vi "Teleop.vi"(10 "Match Info":T1={"Autonomous Elapsed Seconds"=0.0, "TeleOp Elapsed Seconds"=0.0, "Disabled Elapsed Seconds"=0.0, "Visited Autonomous"=FALSE, "Visited TeleOp"=FALSE, "Visited Disabled"=FALSE, "Autonomous Settings"={"Autonomous Style"=enum."Independent", "VI Refnum"=refnum}}, 11 "Call Context":T2) -> ()   [LabVIEW 2013]
doc: "This VI is called for each TeleOp packet received from the DS where the robot is not disabled. It is often used to read from the joysticks and update I/O or to update setpoints for timed control loops. It should complete and return within 20 milliseconds or it may miss DS packets."
uses:
  <vilib>/Rock Robotics/WPI/DriverStation/WPI_DriverStationDerivedRobotMode.ctl
  <vilib>/Rock Robotics/WPI/DriverStation/WPI_DriverStationMatch Info.ctl
  <vilib>/Rock Robotics/WPI/Solenoid/WPI_SolenoidValue.ctl
  Robot Global Data.vi
  <vilib>/Rock Robotics/WPI/RobotDrive/WPI_RobotDriveArcadeDrive_Standard(NoSaturation).vi
  <vilib>/Rock Robotics/WPI/Solenoid/WPI_SolenoidSetEnum.vi
  <vilib>/Rock Robotics/WPI/Joystick/WPI_JoystickGetSetRefNum.vi
  <vilib>/Rock Robotics/WPI/RobotDrive/WPI_RobotDriveGetSetRefNum.vi
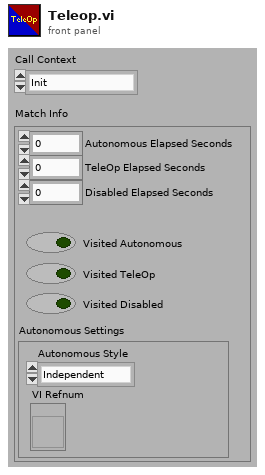
[diagram p1: front panel]
types:
  T1 = typedef "WPI_DriverStationMatch Info.ctl" = cluster{"Autonomous Elapsed Seconds":dbl, "TeleOp Elapsed Seconds":dbl, "Disabled Elapsed Seconds":dbl, "Visited Autonomous":bool, "Visited TeleOp":bool, "Visited Disabled":bool, "Autonomous Settings":cluster{"Autonomous Style":enum16{"Iterative", "Independent"}, "VI Refnum":refnum<vi>}}
  T2 = typedef "WPI_DriverStationDerivedRobotMode.ctl" = enum16{"Init", "Execute", "Stop"}
  T3 = typedef "WPI_SolenoidValue.ctl" = enum16{"Off", "On", "Forward", "Reverse"}
  T4 = typedef "WPI_JoystickDevRef.ctl" = cluster{"Device":T5}
  T5 = typedef "WPI_JoystickDeviceEnum.ctl" = enum16{"USB 1", "USB 2", "USB 3", "USB 4", "Kinect 1", "Kinect 2"}
  T6 = typedef "WPI_MotorControlDeviceRef.ctl" = cluster{"DeviceStatus":errorcluster, "Type":enum16{"PWM", "CAN"}, "PWM":cluster{"Digital Module":T7, "PWM Channel":T8, "DeadBand":T9}, "CAN":cluster{"Device Number":u8, "Control Mode":T10, "Semaphore":T11, "Max Vout":dbl}, "Invert":bool, "TransformRef":T12, "InvTransformRef":T12}
  T7 = typedef "FPGA_TypedefDigitalModule.ctl" = enum16{"Digital Module 1", "Digital Module 2"}
  T8 = typedef "FPGA_DIOPWMChannel.ctl" = enum8{"PWM 1", "PWM 2", "PWM 3", "PWM 4", "PWM 5", "PWM 6", "PWM 7", "PWM 8", "PWM 9", "PWM 10", "Invalid"}
  T9 = typedef "WPI_PWMDeadband.ctl" = cluster{"Name":string, "maxPositivePwm":i32, "minPositivePwm":i32, "centerPwm":i32, "maxNegativePwm":i32, "minNegativePwm":i32, "angularRange":u16}
  T10 = typedef "WPI_CANJaguar_ControlMode.ctl" = enum8{"Percent VBus", "Current", "Speed", "Position", "Voltage"}
  T11 = typedef "Semaphore RefNum" = refnum<k1>
  T12 = typedef "WPI_PWMTransform_ConPane.ctl" = refnum<vi>
  T13 = typedef "WPI_JoystickButtonState.ctl" = cluster{"Button 1":bool, "Button 2":bool, "Button 3":bool, "Button 4":bool, "Button 5":bool, "Button 6":bool, "Button 7":bool, "Button 8":bool, "Button 9":bool, "Button 10":bool, "Button 11":bool, "Button 12":bool}
  T14 = cluster{"axis 1 (x)":dbl, "axis 2 (y)":dbl, "axis 3 (throttle)":dbl, "axis 4":dbl, "axis 5":dbl, "axis 6":dbl}
  T15 = typedef "WPI_SolenoidDevRef.ctl" = cluster{"DevStatus":errorcluster, "Solenoid Module":T16, "Forward Solenoid Channel":T17, "Reverse Solenoid Channel":T17}
  T16 = typedef "FPGA_TypedefSolenoidModule.ctl" = enum16{"Solenoid Module 1", "Solenoid Module 2"}
  T17 = typedef "WPI_SolenoidChannel.ctl" = enum8{"Solenoid 1", "Solenoid 2", "Solenoid 3", "Solenoid 4", "Solenoid 5", "Solenoid 6", "Solenoid 7", "Solenoid 8", "Invalid"}
  T18 = typedef "WPI_RobotDriveDevRef.ctl" = cluster{"DevStatus":errorcluster, "Motors[]":T6[], "Square Inputs":bool, "Max Output":dbl, "Isochronous":bool}
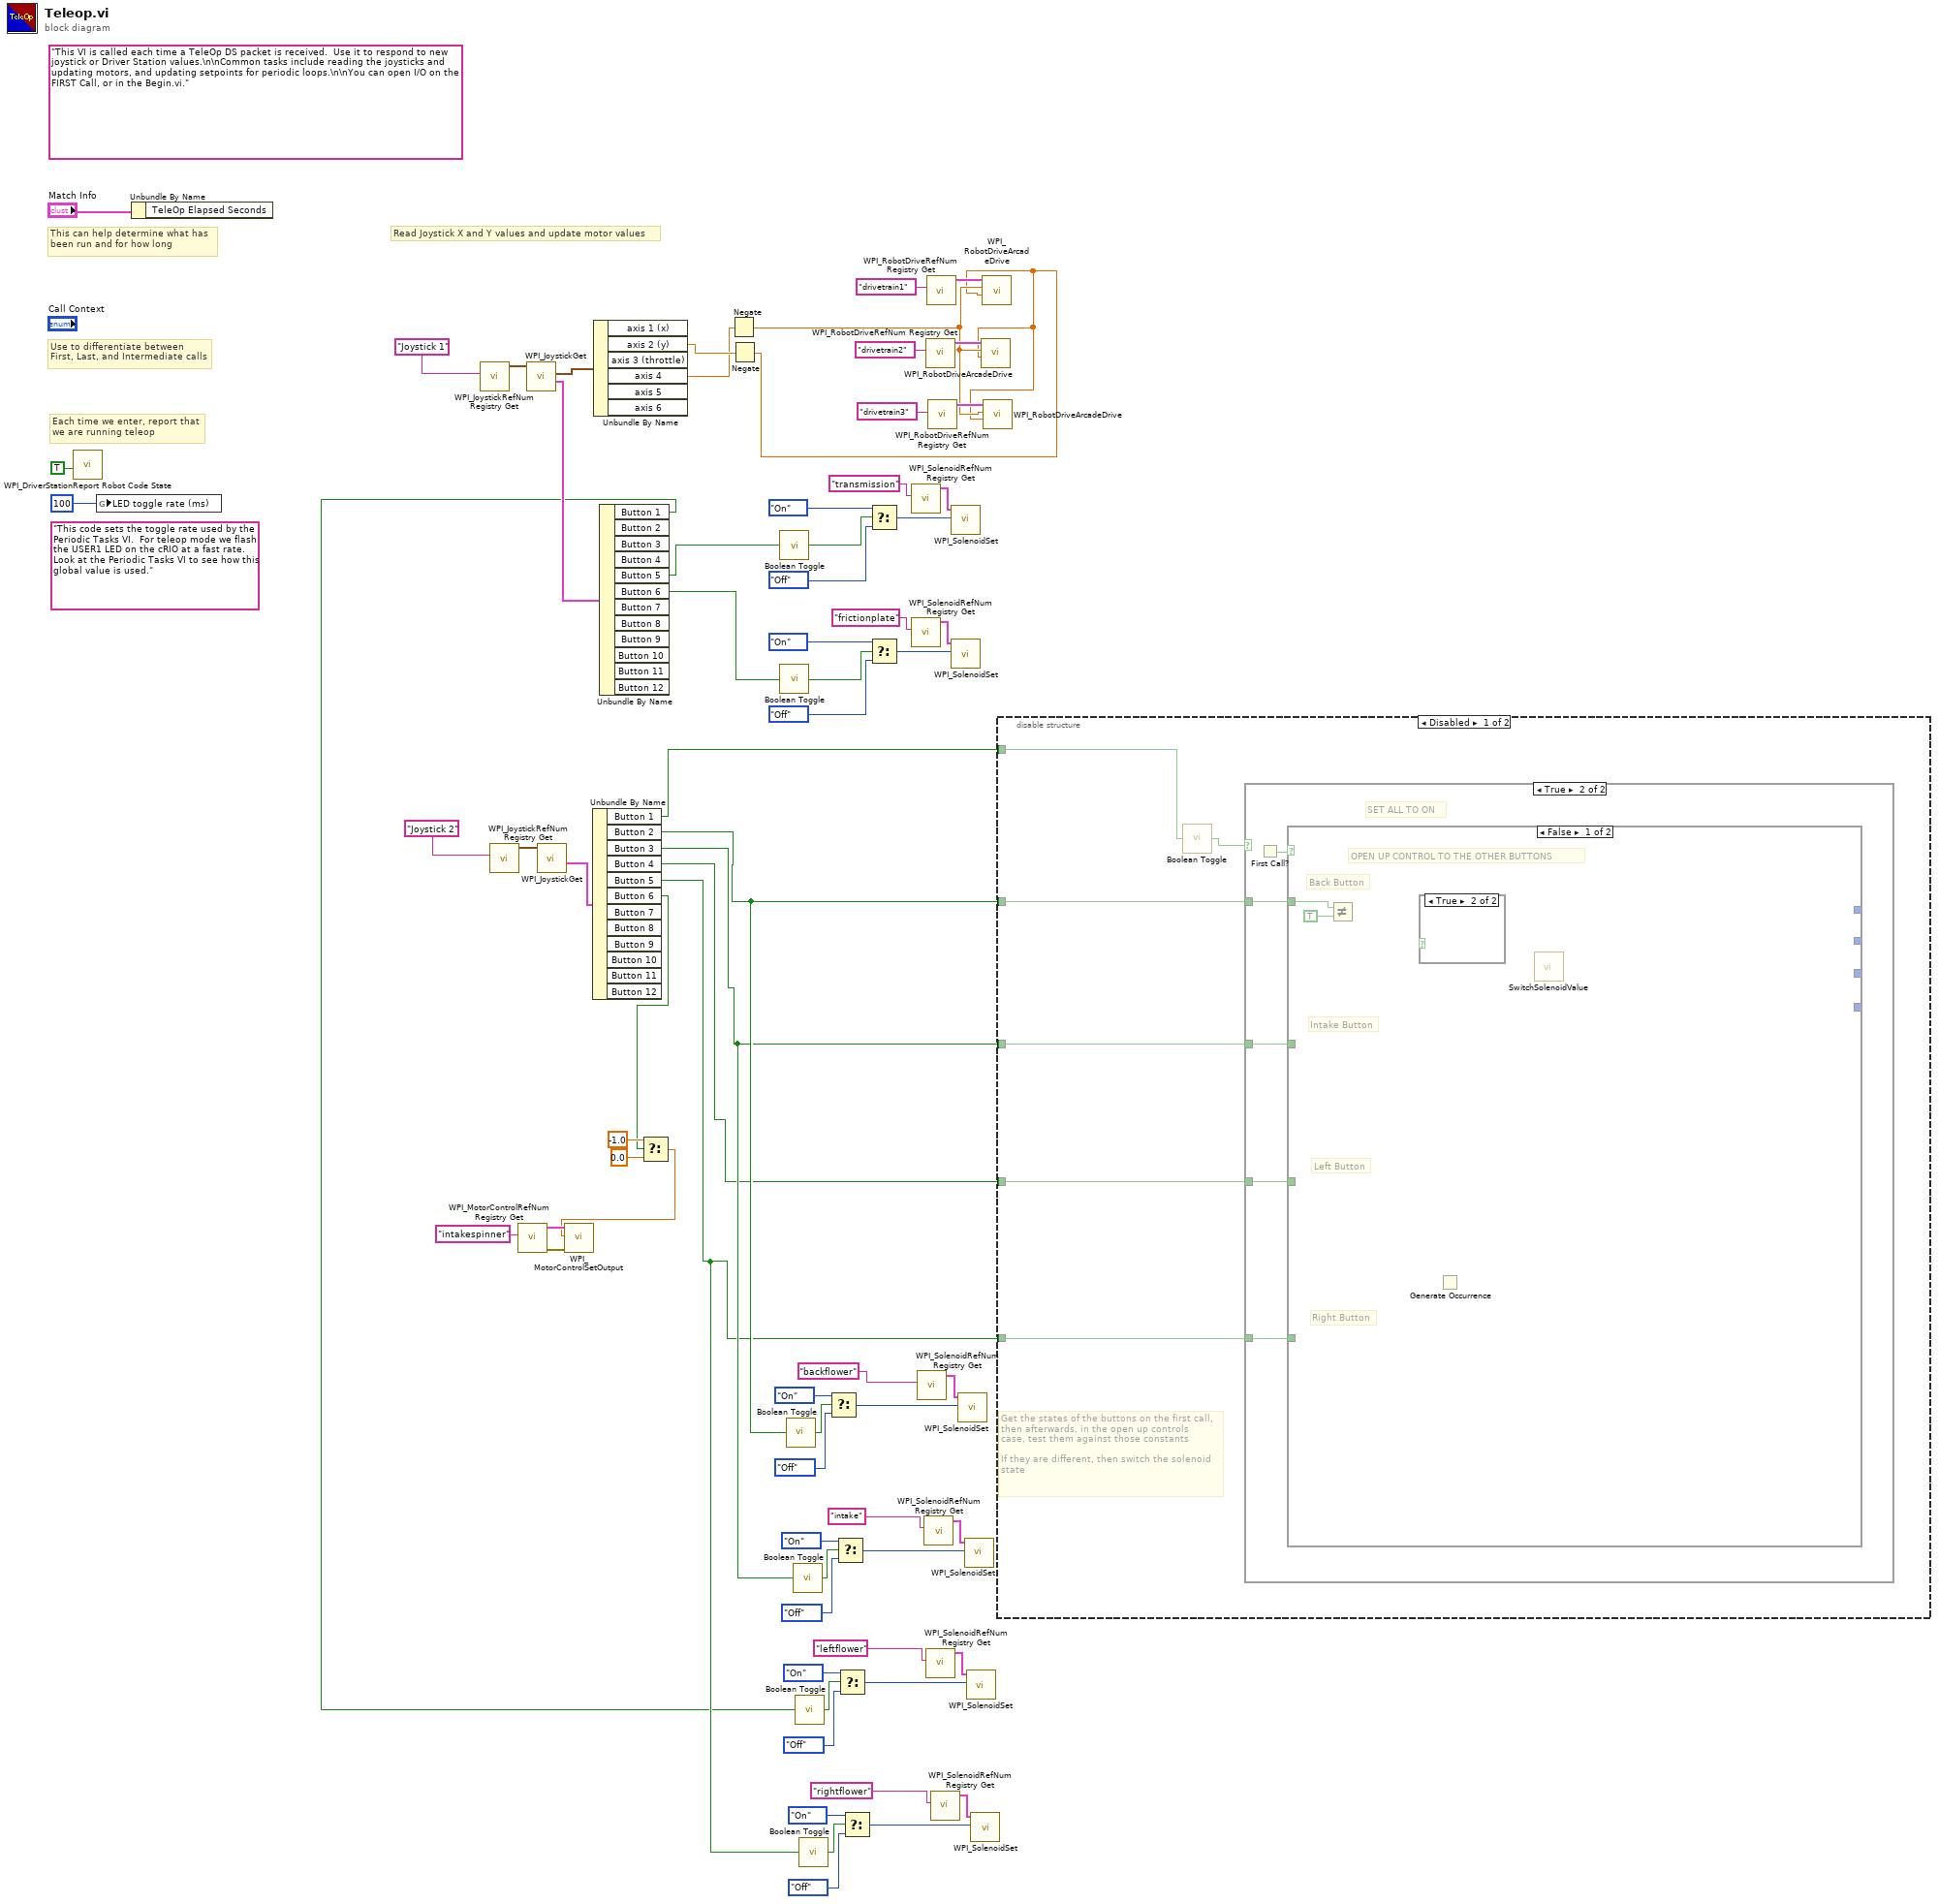
[diagram p0: block diagram]
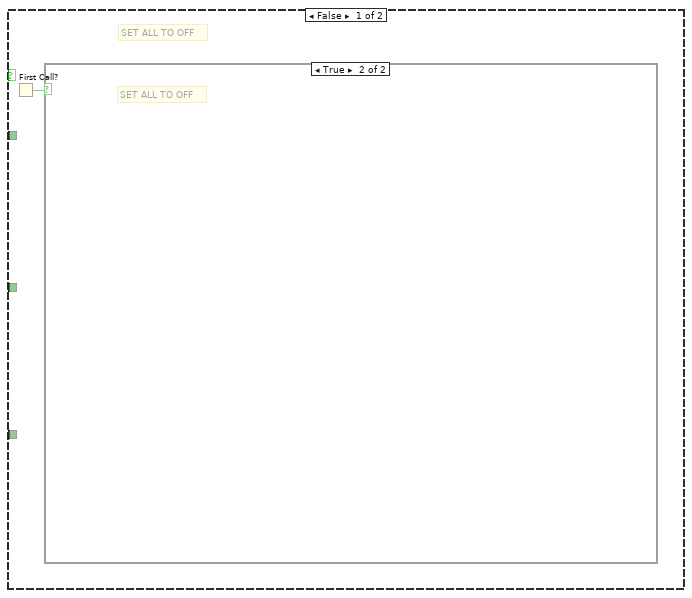
[diagram p2: hidden frame]
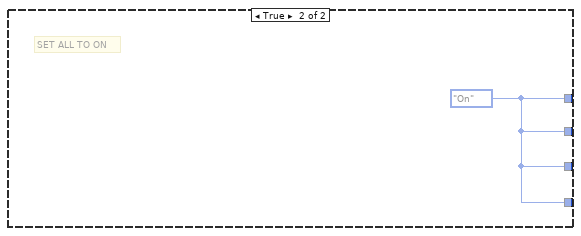
[diagram p5: hidden frame]
diagram:
  (unwired) "This code sets the toggle rate used by the Periodic Tasks VI.  For teleop mode we flash the USER1 LED on the cRIO at a fast rate.  Look at the Periodic Tasks VI to see how this global value is used."
  (unwired) "This VI is called each time a TeleOp DS packet is received.  Use it to respond to new joystick or Driver Station values.\n\nCommon tasks include reading the joysticks and updating motors, and updating setpoints for periodic loops.\n\nYou can open I/O on the FIRST Call, or in the Begin.vi."
  # "Each time we enter, report that\nwe are running teleop"
  # "Use to differentiate between\nFirst, Last, and Intermediate calls"
  # "This can help determine what has\nbeen run and for how long"
  # "Read Joystick X and Y values and update motor values"
  n1 = call <vilib>:"WPI_DriverStationReport Robot Code State.vi"("TeleOp"=TRUE ("Autonomous")) -> ()  [unwired: 10 in, 1 out]
  n2 = global write "Robot Global Data.vi" "LED toggle rate (ms)"(u32 100 ("LED ms toggle rate")) -> ()
  n3 = Unbundle By Name("Match Info") -> ()  [unwired: 1 out]
  n4 = call <vilib>:"WPI_JoystickRefNum Registry Get.vi"("refnum name"="Joystick 1") -> ("JoystickDevRef"=w69:T4)  [unwired: 1 in, 9 out]
  n5 = call <vilib>:"WPI_JoystickRefNum Registry Get.vi"("refnum name"="Joystick 2") -> ("JoystickDevRef"=w39:T4)  [unwired: 1 in, 9 out]
  n6 = call <vilib>:"WPI_MotorControlRefNum Registry Get.vi"("refnum name"="intakespinner") -> ("error out"=w5:errorcluster, "MotorControlDevRef"=w4:T6)  [unwired: 9 in]
  n7 = call <vilib>:"WPI_JoystickGet.vi"("JoystickDevRef"=w69) -> ("Buttons"=w65:T13, "Axes"=w66:T14)  [unwired: 1 in, 4 out]
  n8 = call <vilib>:"WPI_JoystickGet.vi"("JoystickDevRef"=w39) -> ("Buttons"=w38:T13)  [unwired: 1 in, 5 out]
  n9 = Unbundle By Name(w38) -> ("Button 1"=w37:bool, "Button 2"=w12:bool, "Button 3"=w11:bool, "Button 4"=w10:bool, "Button 5"=w9:bool, "Button 6"=w2:bool)  [unwired: 6 out]
  n10 = Unbundle By Name(w66) -> ("axis 2 (y)"=w51:dbl, "axis 4"=w43:dbl)  [unwired: 4 out]
  n11 = Unbundle By Name(w65) -> ("Button 1"=w1:bool, "Button 5"=w42:bool, "Button 6"=w41:bool)  [unwired: 9 out]
  n12 = Select(t=-1.0, s=w2, f=0.0) -> (s? t:f=w3:dbl)
  n13 = call <vilib>:"WPI_MotorControlSetOutput.vi"("error in (no error)"=w5, "Output"=w3, "MotorControlDevRef"=w4) -> ()  [unwired: 6 in, 3 out]
  n14 = Negate(x=w43) -> (-x=w52:dbl)
  n15 = Negate(x=w51) -> (-x=w50:dbl)
  n16 = call "Boolean Toggle.vi"("Input"=w42) -> ("Output"=w55:bool)
  n17 = call "Boolean Toggle.vi"("Input"=w41) -> ("Output"=w46:bool)
  n18 = call "Boolean Toggle.vi"("Input"=w12) -> ("Output"=w15:bool)
  n19 = call "Boolean Toggle.vi"("Input"=w11) -> ("Output"=w27:bool)
  n20 = call "Boolean Toggle.vi"("Input"=w1) -> ("Output"=w21:bool)
  n21 = call "Boolean Toggle.vi"("Input"=w9) -> ("Output"=w33:bool)
  n22 = Select(t=WPI_SolenoidValue."On" ("Value"), s=w15, f=WPI_SolenoidValue."Off" ("Value")) -> (s? t:f=w16:T3)
  n23 = Select(t=WPI_SolenoidValue."On" ("Value"), s=w27, f=WPI_SolenoidValue."Off" ("Value")) -> (s? t:f=w28:T3)
  n24 = Select(t=WPI_SolenoidValue."On" ("Value"), s=w21, f=WPI_SolenoidValue."Off" ("Value")) -> (s? t:f=w22:T3)
  n25 = Select(t=WPI_SolenoidValue."On" ("Value"), s=w33, f=WPI_SolenoidValue."Off" ("Value")) -> (s? t:f=w34:T3)
  n26 = Select(t=WPI_SolenoidValue."On" ("Value"), s=w55, f=WPI_SolenoidValue."Off" ("Value")) -> (s? t:f=w56:T3)
  n27 = Select(t=WPI_SolenoidValue."On" ("Value"), s=w46, f=WPI_SolenoidValue."Off" ("Value")) -> (s? t:f=w47:T3)
  n28 = call <vilib>:"WPI_SolenoidRefNum Registry Get.vi"("refnum name"="transmission") -> ("SolenoidDevRef"=w53:T15)  [unwired: 9 in, 1 out]
  n29 = call <vilib>:"WPI_SolenoidRefNum Registry Get.vi"("refnum name"="frictionplate") -> ("SolenoidDevRef"=w44:T15)  [unwired: 9 in, 1 out]
  n30 = call <vilib>:"WPI_SolenoidRefNum Registry Get.vi"("refnum name"="backflower") -> ("SolenoidDevRef"=w13:T15)  [unwired: 9 in, 1 out]
  n31 = call <vilib>:"WPI_SolenoidRefNum Registry Get.vi"("refnum name"="intake") -> ("SolenoidDevRef"=w25:T15)  [unwired: 9 in, 1 out]
  n32 = call <vilib>:"WPI_RobotDriveRefNum Registry Get.vi"("refnum name"="drivetrain2") -> ("RobotDriveDevRef"=w60:T18)  [unwired: 9 in, 1 out]
  n33 = call <vilib>:"WPI_SolenoidRefNum Registry Get.vi"("refnum name"="leftflower") -> ("SolenoidDevRef"=w19:T15)  [unwired: 9 in, 1 out]
  n34 = call <vilib>:"WPI_RobotDriveRefNum Registry Get.vi"("refnum name"="drivetrain1") -> ("RobotDriveDevRef"=w61:T18)  [unwired: 9 in, 1 out]
  n35 = call <vilib>:"WPI_RobotDriveRefNum Registry Get.vi"("refnum name"="drivetrain3") -> ("RobotDriveDevRef"=w59:T18)  [unwired: 9 in, 1 out]
  n36 = call <vilib>:"WPI_SolenoidRefNum Registry Get.vi"("refnum name"="rightflower") -> ("SolenoidDevRef"=w31:T15)  [unwired: 9 in, 1 out]
  n37 = call-poly <vilib>:"WPI_SolenoidSet.vi"("Value"=w56, "SolenoidDevRef"=w53) -> ()  [unwired: 8 in, 2 out]
  n38 = call-poly <vilib>:"WPI_SolenoidSet.vi"("Value"=w47, "SolenoidDevRef"=w44) -> ()  [unwired: 8 in, 2 out]
  n39 = call-poly <vilib>:"WPI_SolenoidSet.vi"("Value"=w16, "SolenoidDevRef"=w13) -> ()  [unwired: 8 in, 2 out]
  n40 = call-poly <vilib>:"WPI_SolenoidSet.vi"("Value"=w28, "SolenoidDevRef"=w25) -> ()  [unwired: 8 in, 2 out]
  n41 = call-poly <vilib>:"WPI_SolenoidSet.vi"("Value"=w22, "SolenoidDevRef"=w19) -> ()  [unwired: 8 in, 2 out]
  n42 = call-poly <vilib>:"WPI_SolenoidSet.vi"("Value"=w34, "SolenoidDevRef"=w31) -> ()  [unwired: 8 in, 2 out]
  n43 = call-poly <vilib>:"WPI_RobotDriveArcadeDrive.vi"("Y axis value"=w50, "X axis value"=w52, "RobotDriveDevRef"=w60) -> ()  [unwired: 6 in, 3 out]
  n44 = call-poly <vilib>:"WPI_RobotDriveArcadeDrive.vi"("Y axis value"=w50, "X axis value"=w52, "RobotDriveDevRef"=w61) -> ()  [unwired: 6 in, 3 out]
  n45 = call-poly <vilib>:"WPI_RobotDriveArcadeDrive.vi"("Y axis value"=w50, "X axis value"=w52, "RobotDriveDevRef"=w59) -> ()  [unwired: 6 in, 3 out]
  n46 = disable-structure shown="Disabled" {
    disable-tunnel: w37 -> [w76 _]
    disable-tunnel: w12 -> [w75 _]
    disable-tunnel: w11 -> [w74 _]
    disable-tunnel: w10 -> [w73 _]
    disable-tunnel: w9 -> [w72 _]
    frame Disabled {
      # "Get the states of the buttons on the first call,\nthen afterwards, in the open up controls\ncase, test them against those constants\n\nIf they are different, then switch the solenoid\nstate"
      n47 = call "Boolean Toggle.vi"("Input"=w76) -> ("Output"=w77:bool)
      n48 = case shown="True" w77 {
        tunnel: w75 -> [_ w82]
        tunnel: w74 -> [_ w81]
        tunnel: w73 -> [_ w80]
        tunnel: w72 -> [_ w79]
        frame False {
          # "SET ALL TO OFF"
          n49 = First Call?() -> (First Call?: T/F=w78:bool)
          n50 = case shown="True" w78 {
            frame False {
            }
            frame True {
              # "SET ALL TO OFF"
            }
          }
        }
        frame True {
          # "SET ALL TO ON"
          n51 = First Call?() -> (First Call?: T/F=w83:bool)
          n52 = case shown="False" w83 {
            tunnel: [_ w86] -> _
            tunnel: [_ w86] -> _
            tunnel: [_ w86] -> _
            tunnel: [_ w86] -> _
            tunnel: w82 -> [w85 _]
            tunnel: w81 -> [_ _]
            tunnel: w80 -> [_ _]
            tunnel: w79 -> [_ _]
            frame False {
              # "Right Button"
              # "Left Button"
              # "Intake Button"
              # "Back Button"
              # "OPEN UP CONTROL TO THE OTHER BUTTONS"
              n53 = Not Equal?(x=w85, y=TRUE) -> ()  [unwired: 1 out]
              n54 = case shown="True" {
                selector: _ -> [_ _]
                frame False {
                }
                frame True {
                }
              }
              n55 = Generate Occurrence() -> ()  [unwired: 1 out]
              n56 = call "SwitchSolenoidValue.vi"() -> ()  [unwired: 2 in, 1 out]
            }
            frame True {
              w86 = WPI_SolenoidValue."On" ("Value")
              # "SET ALL TO ON"
            }
          }
        }
      }
    }
    frame Enabled {
    }
  }
